vi "GNSS Read.vi"(8 "Measurement In":refnum<data-value>, 10 "GNSS Handle":T1, 11 "Error In":errorcluster) -> (0 "Measurement Out":refnum<data-value>, 1 "GNSS Data":T2, 3 "Error Out":errorcluster)   [LabVIEW 2021]
uses:
  GNSS Data.ctl
  GNSS Handle.ctl
  State Estimator/Measurements.ctl
  IMU/IMU Data.ctl
  Steering Motor Encoder/Steering Motor Encoder Data.ctl
panel:
  out "time":string
  out "status":string
  out "x+1":u32
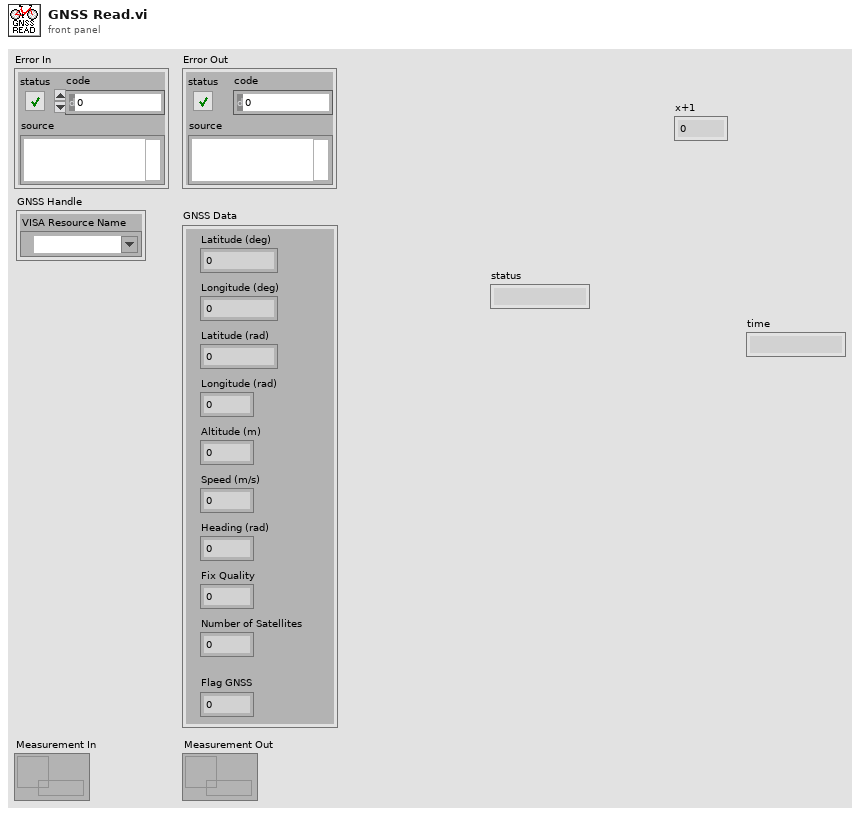
[diagram p1: front panel]
types:
  T1 = typedef "GNSS Handle.ctl" = cluster{"VISA Resource Name":refnum<visa-resource-name>}
  T2 = typedef "GNSS Data.ctl" = cluster{"Latitude (rad)":dbl, "Longitude (rad)":dbl, "Altitude (m)":dbl, "Speed (m/s)":dbl, "Heading (rad)":dbl, "Fix Quality":i32, "Number of Satellites":i32, "Latitude (deg)":dbl, "Longitude (deg)":dbl, "Flag GNSS":dbl}
  T3 = typedef "Measurements.ctl" = cluster{"IMU Data":T4, "Steering Motor Encoder Data":T5, "GNSS Data":T2}
  T4 = typedef "IMU Data.ctl" = cluster{"Gyroscope":cluster{"X (rad/s)":dbl, "Y (rad/s)":dbl, "Z (rad/s)":dbl}, "Accelerometer":cluster{"X (m/s^2)":dbl, "Y (m/s^2)":dbl, "Z (m/s^2)":dbl}, "Flag IMU":dbl}
  T5 = typedef "Steering Motor Encoder Data.ctl" = cluster{"Encoder Position (counts)":i32, "Steering Angle (rad)":dbl, "Flag Steering Encoder":dbl}
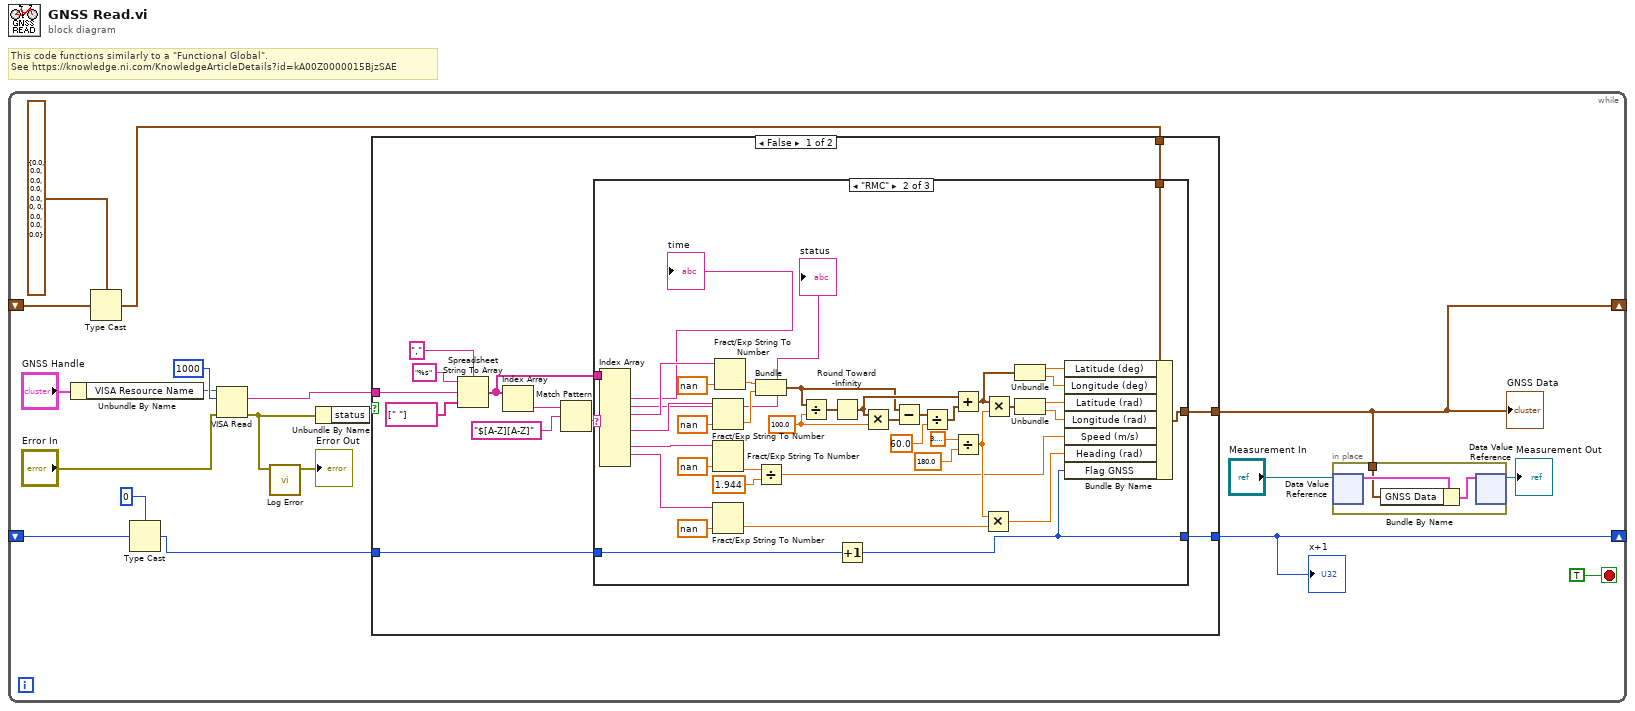
[diagram p0: block diagram]
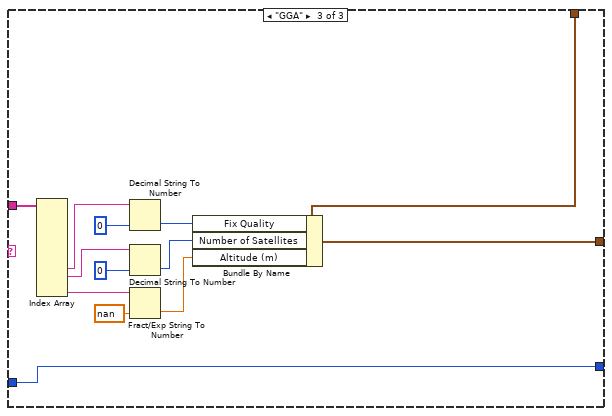
[diagram p3: hidden frame]
diagram:
  # "This code functions similarly to a \"Functional Global\".\nSee https://knowledge.ni.com/KnowledgeArticleDetails?id=kA00Z0000015BjzSAE"
  n1 = while {
    shift-right: [w8] -> _
    shift-left: _ -> [w7]
    shift-right: [w1] -> _
    shift-left: _ -> [w2]
    stop <- TRUE stop-if-true
    n2 = Unbundle By Name("GNSS Handle") -> ("VISA Resource Name"=w15:refnum<visa-resource-name>)
    n3 = Type Cast(type=T2 {"Latitude (rad)"=0.0, "Longitude (rad)"=0.0, "Altitude (m)"=0.0, "Speed (m/s)"=0.0, "Heading (rad)"=0.0, "Fix Quality"=0, "Number of Satellites"=0, "Latitude (deg)"=0.0, "Longitude (deg)"=0.0, "Flag GNSS"=0.0} ("GNSS Data 2"), x=w7) -> (*(type *) &x=w6:T2)
    n4 = Type Cast(type=u32 0 ("byte count"), x=w2) -> (*(type *) &x=w3:u32)
    n5 = VISA Read(VISA resource name=w15, byte count=u32 1000, error in (no error)="Error In") -> (read buffer=w18:string, error out=w10:errorcluster)  [unwired: 2 out]
    n6 = call "Log Error.vi"("Error In"=w10) -> ("Error Out"=→"Error Out":errorcluster)  [unwired: 10 in]
    n7 = Unbundle By Name(w10) -> ("status"=w19:bool)
    n8 = case shown="False" w19 {
      tunnel: w18 -> [w34 _]
      tunnel: w6 -> [w26 w90]
      tunnel: [w25 w90] -> w8
      tunnel: w3 -> [w24 w89]
      tunnel: [w23 w89] -> w1
      frame False {
        n9 = Spreadsheet String To Array(delimiter (Tab)=",", format string="%s", spreadsheet string=w34, array type (2D Dbl)=string[] [" "]) -> (array=w27:string[])
        n10 = Index Array(array=w27) -> (element=w30:string)  [unwired: 1 in]
        n11 = Match Pattern(string=w30, regular expression="$[A-Z][A-Z]") -> (after substring=w28:string)  [unwired: 1 in, 3 out]
        n12 = case shown="\"RMC\"" w28 {
          tunnel: w27 -> [_ w75 w88]
          tunnel: w26 -> [w36 w46 w78]
          tunnel: [w36 w45 w77] -> w25
          tunnel: w24 -> [w35 w40 w76]
          tunnel: [w35 w39 w76] -> w23
          frame Default {
          }
          frame "RMC" {
            w68 = 100.0 ("y")
            n13 = Index Array(array=w75) -> (element #2=→"time":string, element #3=→"status":string, element #4=w50:string, element #6=w72:string, element #8=w58:string, element #9=w53:string)  [unwired: 10 in, 4 out]
            n14 = Fract/Exp String To Number(string=w72, default (0 dbl)=nan ("default (0 DBL)")) -> (number=w71:dbl)  [unwired: 2 in, 1 out]
            n15 = Fract/Exp String To Number(string=w58, default (0 dbl)=nan ("default (0 DBL)")) -> (number=w57:dbl)  [unwired: 2 in, 1 out]
            n16 = Fract/Exp String To Number(string=w53, default (0 dbl)=nan ("default (0 DBL)")) -> (number=w52:dbl)  [unwired: 2 in, 1 out]
            n17 = Fract/Exp String To Number(string=w50, default (0 dbl)=nan ("default (0 DBL)")) -> (number=w70:dbl)  [unwired: 2 in, 1 out]
            n18 = Bundle(w70, w71) -> (w62:cluster{dbl, dbl})  [unwired: 1 in]
            n19 = Divide(x=w57, y=1.944) -> (x/y=w47:dbl)
            n20 = Divide(x=w62, y=w68) -> (x/y=w69:cluster{dbl, dbl})
            n21 = Round Toward -Infinity(1:w69) -> (0:w64:cluster{dbl, dbl})
            n22 = Increment(x=w40) -> (x+1=w39:u32)
            n23 = Multiply(x=w64, y=w68) -> (x*y=w67:cluster{dbl, dbl})
            n24 = Subtract(x=w62, y=w67) -> (x-y=w65:cluster{dbl, dbl})
            n25 = Divide(x=w65, y=60.0) -> (x/y=w63:cluster{dbl, dbl})
            n26 = Add(x=w64, y=w63) -> (x+y=w41:cluster{dbl, dbl})
            n27 = Divide(x=3.141592653589793, y=180.0) -> (x/y=w51:dbl)
            n28 = Multiply(x=w51, y=w52) -> (x*y=w48:dbl)
            n29 = Multiply(x=w41, y=w51) -> (x*y=w59:cluster{dbl, dbl})
            n30 = Unbundle(w41) -> (w43:dbl, w42:dbl)
            n31 = Unbundle(w59) -> (w44:dbl, w49:dbl)
            n32 = Bundle By Name(cluster=w46, "Latitude (deg)"=w43, "Longitude (deg)"=w42, "Latitude (rad)"=w44, "Longitude (rad)"=w49, "Speed (m/s)"=w47, "Heading (rad)"=w48, "Flag GNSS"=w39) -> (w45:T2)
          }
          frame "GGA" {
            n33 = Index Array(array=w88) -> (element #7=w87:string, element #8=w86:string, element #10=w85:string)  [unwired: 10 in, 7 out]
            n34 = Decimal String To Number(string=w87, default (0L)=0 ("default (0 I32)")) -> (number=w81:i32)  [unwired: 1 in, 1 out]
            n35 = Decimal String To Number(string=w86, default (0L)=0 ("default (0 I32)")) -> (number=w80:i32)  [unwired: 1 in, 1 out]
            n36 = Fract/Exp String To Number(string=w85, default (0 dbl)=nan ("default (0 DBL)")) -> (number=w79:dbl)  [unwired: 2 in, 1 out]
            n37 = Bundle By Name(cluster=w78, "Fix Quality"=w81, "Number of Satellites"=w80, "Altitude (m)"=w79) -> (w77:T2)
          }
        }
      }
      frame True {
      }
    }
    "GNSS Data" <- w8
    "x+1" <- w1
    n38 = in-place {
      in-place-border: w8 -> [w20]
      n39 = in-place-dvr #1("Measurement In") -> (w22:T3)  [unwired: 1 out]
      n40 = Bundle By Name(cluster=w22, "GNSS Data"=w20) -> (w21:T3)
      n41 = in-place-dvr #1(w21) -> (→"Measurement Out":refnum<data-value>)  [unwired: 1 out]
    }
  }
